vi "CTRE_Phoenix_CANdle_GetStatusFramePeriod.vi"(6 "timeoutMs":u32, 8 "error in":errorcluster, 10 "CANdle Status Frame":T1=267264 items=["Status_1_General"=267264, "Status_2_Startup"=267328, "Status_3_FirmwareApiStatus"=267392, "Status_4_ControlTelem"=267456, "Status_5_PixelPulseTrain"=267520, "Status_6_BottomPixels"=267584, "Status_7_TopPixels"=267648], 11 "CTRE_CANdle_DeviceRef":T2) -> (0 "error out":errorcluster, 2 "periodMs":u32, 3 "CTRE_CANdle_DeviceRef":T2)   [LabVIEW 2020]
doc: "Returns the period of the selected Status Frame."
uses:
  <vilib>/Rock Robotics/WPI/ThirdParty/Phoenix-LabVIEW/CANdle/Controls/CTRE_Phoenix_CANdle_DeviceRef.ctl
  <vilib>/Rock Robotics/WPI/ThirdParty/Phoenix-LabVIEW/CANdle/Controls/CTRE_Phoenix_CANdle_StatusFrame.ctl
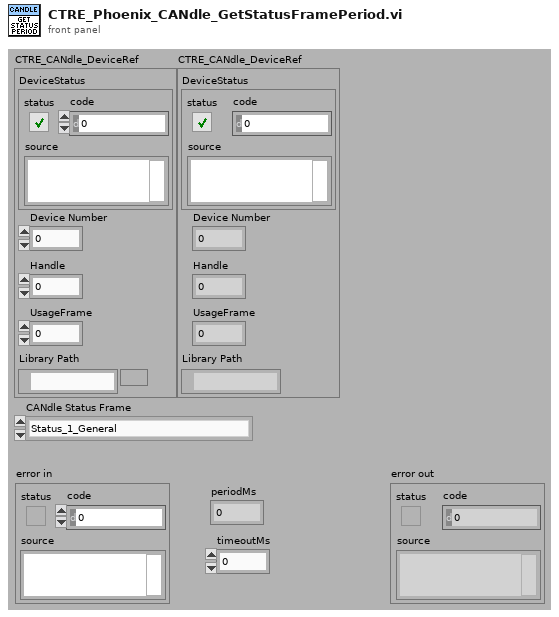
[diagram p1: front panel]
types:
  T1 = typedef "CTRE_Phoenix_CANdle_StatusFrame.ctl" = u32
  T2 = typedef "CTRE_Phoenix_CANdle_DeviceRef.ctl" = cluster{"DeviceStatus":errorcluster, "Device Number":u8, "Handle":u64, "UsageFrame":u32, "Library Path":path}
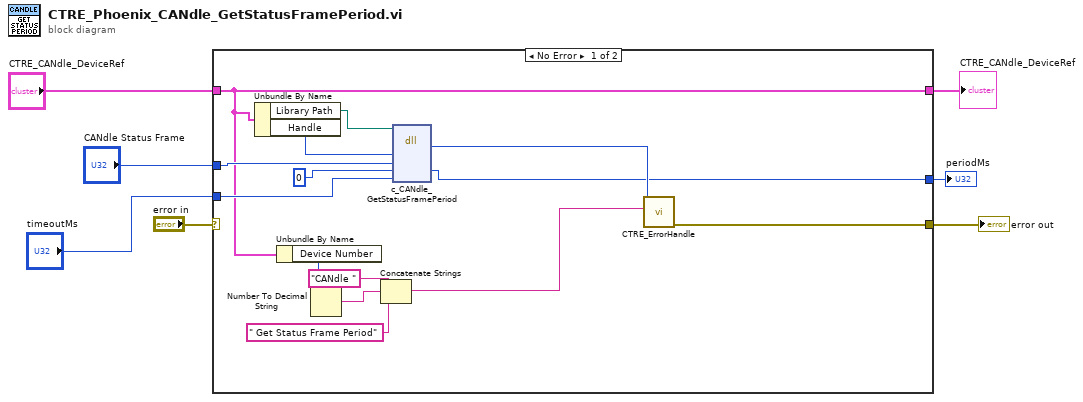
[diagram p0: block diagram]
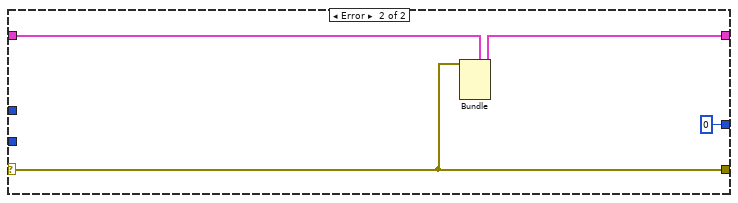
[diagram p2: hidden frame]
diagram:
  n1 = case shown="No Error" "error in" {
    selector: "error in" -> [_ w24]
    tunnel: "CTRE_CANdle_DeviceRef" -> [w10 w25]
    tunnel: [w20 w24] -> w7
    tunnel: [w10 w23] -> w2
    tunnel: [w13 0 ("percentOutput")] -> w5
    tunnel: "timeoutMs" -> [w12 _]
    tunnel: "CANdle Status Frame" -> [w11 _]
    frame No Error {
      n2 = Unbundle By Name(w10) -> ("Library Path"=w9:path, "Handle"=w8:u64)
      n3 = Unbundle By Name(w10) -> ("Device Number"=w16:u8)
      n4 = Number To Decimal String(number=w16) -> (decimal integer string=w18:string)  [unwired: 1 in]
      n5 = Concatenate Strings("CANdle " ("string"), w18, " Get Status Frame Period" ("string")) -> (w14:string)
      n6 = dll-call lib="?" fn="c_CANdle_GetStatusFramePeriod"(path in=w9, "handle"=w8, "frame"=w11, "periodMs"=u32 0 ("appliedThrottle"), "timeoutMs"=w12) -> ("return type"=w15:i32, "periodMs"=w13:u32)  [unwired: 5 in, 2 out]
      n7 = call <vilib>:"CTRE_ErrorHandle.vi"("origin"=w14, "code"=w15) -> ("error out"=w20:errorcluster)  [unwired: 9 in]
    }
    frame Error {
      n8 = Bundle(cluster=w25, "DeviceStatus"=w24) -> (w23:T2)  [unwired: 4 in]
    }
  }
  "error out" <- w7
  "periodMs" <- w5
  "CTRE_CANdle_DeviceRef" <- w2
